vi "Stop_cycle.vi"(11 "Refs cluster In":T1) -> (5 "Stop?":bool)   [LabVIEW 2015]
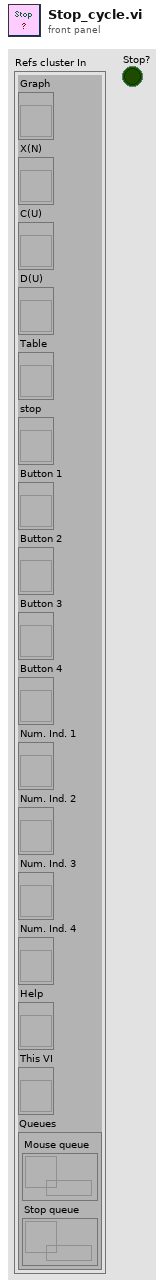
[diagram p1: front panel]
types:
  T1 = cluster{"Graph":refnum<vi>, "X(N)":refnum<vi>, "C(U)":refnum<vi>, "D(U)":refnum<vi>, "Table":refnum<vi>, "stop":refnum<vi>, "Button 1":refnum<vi>, "Button 2":refnum<vi>, "Button 3":refnum<vi>, "Button 4":refnum<vi>, "Num. Ind. 1":refnum<vi>, "Num. Ind. 2":refnum<vi>, "Num. Ind. 3":refnum<vi>, "Num. Ind. 4":refnum<vi>, "Help":refnum<vi>, "This VI":refnum<vi>, "Queues":cluster{"Mouse queue":refnum<queue>, "Stop queue":refnum<queue>}}
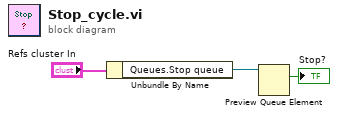
[diagram p0: block diagram]
diagram:
  n1 = Unbundle By Name("Refs cluster In") -> ("Queues.Stop queue"=w2:refnum<queue>)
  n2 = Preview Queue Element(queue=w2) -> (element=→"Stop?":bool)  [unwired: 2 in, 3 out]
